vi "adcexo2.vi"() -> ()   [LabVIEW 2020]
uses:
  <vilib>/Analysis/baseanly.llb/Mean (DBL).vi
  <vilib>/Analysis/NI_AALBase.lvlib
panel:
  out "without shift":dynamicdata(graph)
  out "mean":dbl format="%0.2f"
  out "aquired":dynamicdata(graph)
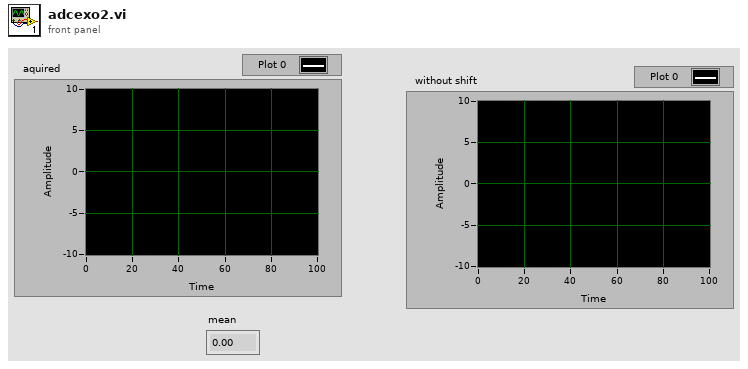
[diagram p1: front panel]
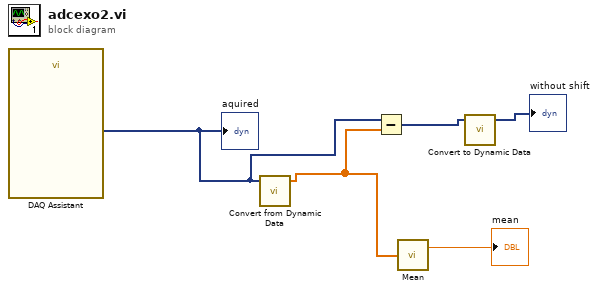
[diagram p0: block diagram]
diagram:
  n1 = call "DAQ Assistant"() -> ("data"=w4:dynamicdata)  [unwired: 17 in, 2 out]
  "aquired" <- w4
  n2 = call "Convert from Dynamic Data"("Dynamic Data Type"=w4) -> ("Array"=w3:dbl[])  [unwired: 3 in]
  n3 = Subtract(x=w4, y=w3) -> (x-y=w2:dynamicdata[])
  n4 = call-poly <vilib>:"Mean.vi"("X"=w3) -> ("mean"=→"mean":dbl)  [unwired: 1 out]
  n5 = call "Convert to Dynamic Data"("Array of Waveforms"=w2) -> ("Dynamic Data Type"=→"without shift":dynamicdata)  [unwired: 3 in]
